vi "Flatten FIFO Config.vi"(8 "error in":errorcluster, 10 "Flattened Data in":u8[](array[numeric])=[0, 0, 0, 0, 0, 0, 0, 0, 0, 0, 0, 0, 0, 0, 0, 0], 11 "FIFO Config in":T1) -> (0 "error out":errorcluster, 2 "Flattened Data out":u8[](array[numeric]), 3 "FIFO Config out":T1)   [LabVIEW 2021, in "ChannelCommon.lvlib"]
uses:
  ChannelCommon.lvlib
  CIFCore/Common/CIFCoreCommon.lvlib
  CIFUtilities/CIFClocks/Typedef/Errors.ctl
  typedef/FIFO Config.ctl
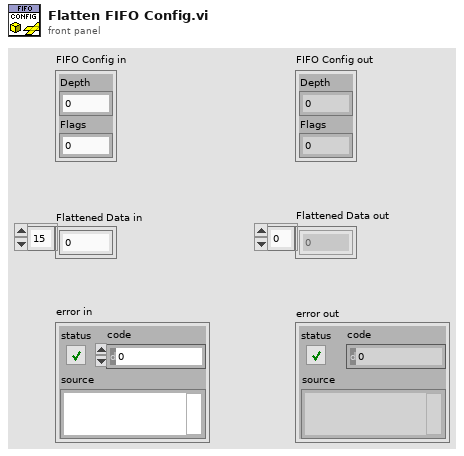
[diagram p1: front panel]
types:
  T1 = typedef "ChannelCommon.lvlib/FIFO Config.ctl" = cluster{"Depth":u64, "Flags":u64}
  T2 = typedef "CIFCoreCommon.lvlib/Errors.ctl" = enum16{"Invalid Clock ID", "Long Sleep", "gRPC Server Not Found", "Config Parse", "Timestamp Wrap", "Delayed Execution", "Duplicate Channel", "Missing Channel", "Incorrect Type", "Flatten Error"}
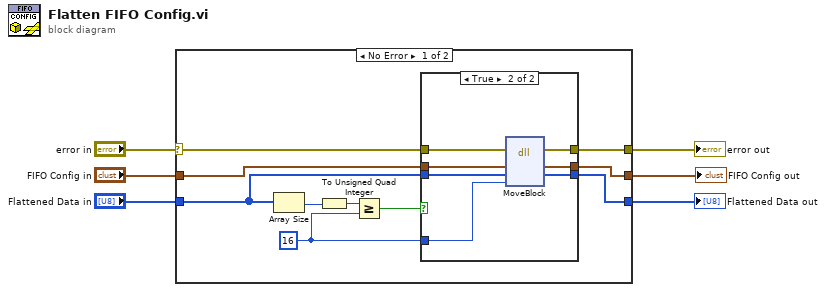
[diagram p0: block diagram]
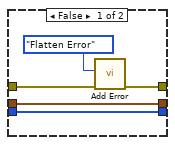
[diagram p2: hidden frame]
diagram:
  n1 = case shown="No Error" "error in" {
    selector: "error in" -> [w7 w31]
    tunnel: "FIFO Config in" -> [w16 w30]
    tunnel: [w15 w31] -> w5
    tunnel: [w14 w29] -> w4
    tunnel: [w13 w30] -> w1
    tunnel: "Flattened Data in" -> [w12 w29]
    frame No Error {
      w10 = u64 16 ("size")
      n2 = Array Size(array=w12) -> (size(s)=w11:i32)
      n3 = To Unsigned Quad Integer(1:w11) -> (0:w9:u64)
      n4 = Greater Or Equal?(x=w9, y=w10) -> (x >= y?=w8:bool)
      n5 = case shown="True" w8 {
        tunnel: w7 -> [w19 w28]
        tunnel: w16 -> [w20 w27]
        tunnel: [w18 w26] -> w15
        tunnel: [w21 w25] -> w14
        tunnel: [w20 w24] -> w13
        tunnel: w12 -> [w21 w23]
        tunnel: w10 -> [_ w22]
        frame False {
          n6 = call "Add Error.vi"("error in (no error)"=w19, "Error"=Errors."Flatten Error") -> ("error out"=w18:errorcluster)  [unwired: 9 in]
        }
        frame True {
          n7 = dll-call lib="LabVIEW" fn="MoveBlock"(error in=w28, "source"=w27, "dest"=w23, "size"=w22) -> (error out=w26:errorcluster, "source"=w24:T1, "dest"=w25:u8[])  [unwired: 4 in, 1 out]
        }
      }
    }
    frame Error {
    }
  }
  "error out" <- w5
  "Flattened Data out" <- w4
  "FIFO Config out" <- w1
